vi "COMTRADE Read Data.vi"(0 "task in":T3={"file refnums"=[], "Data Object"=refnum, "config info"={"station_name"="", "rec_dev_id"="", "rev_year"=1999.0, "TT"=0, "##A"=0, "##D"=0, "analog channel info"=[], "status channel info"=[], "lf"=50.0, "nrates"=0, "samp info"=[], "initial timestamp"=timestamp(0 s since 1904-01-01), "trigger timestamp"=timestamp(0 s since 1904-01-01), "ft"=enum."Binary", "timemult"=1.0}, "public inf content"={"Source"="", "Record Type"=enum."Unknown", "Phase ID"="", "Event Description"="", "Device ID"="", "Distance of Fault"=-1.0, "Distance Unit"=enum."Miles", "Max_Current"=inf, "Min_Current"=-inf, "Max_Voltage"=inf, "Min_Voltage"=-inf, "EventNoteCount"=0, "Event Information"=[]}, "private inf content"=[], "internal buffers"={"start index"=1, "config to public inf"=enum."disabled", "static config info"="", "static file_des record inf"="", "static file_des channel inf"="", "public inf"="", "private inf"=""}} {"public inf content"."Event Information"."min sample number" max=9999999999; "public inf content"."Event Information"."max sample number" max=9999999999; "config info"."nrates" max=999; "config info"."status channel info"."Dn" min=1 max=999999; "config info"."analog channel info"."An" min=1 max=999999; "config info"."trigger timestamp" format="%<%H:%M:%S%6u\n%d/%m/%Y>T"; "config info"."initial timestamp" format="%<%H:%M:%S%6u\n%d/%m/%Y>T"; "config info"."##D" max=999999; "config info"."##A" max=999999; "config info"."TT" min=1 max=999999; "config info"."rev_year" min=1999.0 max=1999.0}, 11 "error in (no error)":errorcluster) -> (3 "number of sample rates":i32 min=0 max=999, 4 "task out":T3={"file refnums"=[], "Data Object"=refnum, "config info"={"station_name"="", "rec_dev_id"="", "rev_year"=1999.0, "TT"=0, "##A"=0, "##D"=0, "analog channel info"=[], "status channel info"=[], "lf"=50.0, "nrates"=0, "samp info"=[], "initial timestamp"=timestamp(0 s since 1904-01-01), "trigger timestamp"=timestamp(0 s since 1904-01-01), "ft"=enum."Binary", "timemult"=1.0}, "public inf content"={"Source"="", "Record Type"=enum."Unknown", "Phase ID"="", "Event Description"="", "Device ID"="", "Distance of Fault"=-1.0, "Distance Unit"=enum."Miles", "Max_Current"=inf, "Min_Current"=-inf, "Max_Voltage"=inf, "Min_Voltage"=-inf, "EventNoteCount"=0, "Event Information"=[]}, "private inf content"=[], "internal buffers"={"start index"=1, "config to public inf"=enum."disabled", "static config info"="", "static file_des record inf"="", "static file_des channel inf"="", "public inf"="", "private inf"=""}} {"public inf content"."Event Information"."min sample number" max=9999999999; "public inf content"."Event Information"."max sample number" max=9999999999; "config info"."nrates" max=999; "config info"."status channel info"."Dn" min=1 max=999999; "config info"."analog channel info"."An" min=1 max=999999; "config info"."trigger timestamp" format="%<%H:%M:%S%6u\n%d/%m/%Y>T"; "config info"."initial timestamp" format="%<%H:%M:%S%6u\n%d/%m/%Y>T"; "config info"."##D" max=999999; "config info"."##A" max=999999; "config info"."TT" min=1 max=999999; "config info"."rev_year" min=1999.0 max=1999.0}, 6 "sample rate information":T2(array[cluster]), 8 "analog data":T1(array[cluster]), 10 "digital data":digitaldata, 14 "timestamps":timestamp[](array[timestamp]), 15 "error out":errorcluster)   [LabVIEW 2014, in "NI_EP_COMTRADE.lvlib"]
doc: "Reads analog data and digital data from the specified .dat file. You must set <B>open mode</B> to Open (read only) in the COMTRADE Open VI to open the .inf file. Otherwise this VI returns an error."
uses:
  <vilib>/addons/Electrical Power/File IO/NI_EP_COMTRADE.lvlib
  <vilib>/addons/Electrical Power/File IO/COMTRADE/typedefs/ep_Task.ctl
  <vilib>/addons/Electrical Power/File IO/COMTRADE/typedefs/ep_Config Info.ctl
  <vilib>/addons/Electrical Power/File IO/COMTRADE/typedefs/ep_Analog Channel Info.ctl
  <vilib>/addons/Electrical Power/File IO/COMTRADE/typedefs/ep_Status Channel Info.ctl
  <vilib>/addons/Electrical Power/File IO/COMTRADE/typedefs/ep_File Format.ctl
  <vilib>/addons/Electrical Power/File IO/COMTRADE/typedefs/ep_Public Inf Content.ctl
  <vilib>/addons/Electrical Power/File IO/COMTRADE/typedefs/ep_Public Event Inf.ctl
  <vilib>/addons/Electrical Power/File IO/COMTRADE/typedefs/ep_Private Inf Content.ctl
  <vilib>/Analysis/1siggen.llb/Ramp Pattern by Samples.vi
  <vilib>/Platform/storage/Storage.llb/Get Property (Storage Refnums).vi
  <vilib>/Platform/storage/Storage.llb/Get Property (I32).vi
  <vilib>/Platform/storage/Storage.llb/Get Property (String).vi
  <vilib>/Platform/storage/Storage.llb/Get Property (SGL).vi
  <vilib>/Waveform/DTblOps.llb/DTbl Boolean Array to Digital.vi
  <vilib>/Analysis/NI_AALBase.lvlib
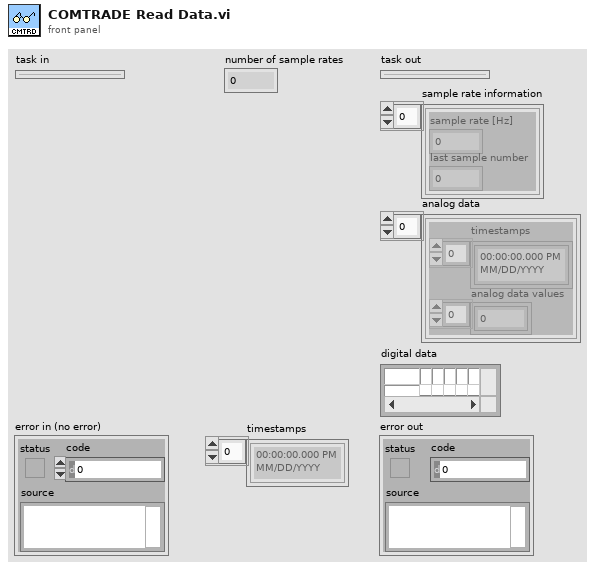
[diagram p1: front panel]
types:
  T1 = cluster{"timestamps":timestamp[], "analog data values":sgl[]}[]
  T2 = cluster{"sample rate [Hz]":sgl, "last sample number":u32}[]
  T3 = typedef "NI_EP_COMTRADE.lvlib/ep_Task.ctl" = cluster{"file refnums":refnum<file>[], "Data Object":refnum<k20>, "config info":T4, "public inf content":T8, "private inf content":T10, "internal buffers":cluster{"start index":u32, "config to public inf":enum16{"disabled", "enabled", "buffered"}, "static config info":string, "static file_des record inf":string, "static file_des channel inf":string, "public inf":string, "private inf":string}}
  T4 = typedef "NI_EP_COMTRADE.lvlib/ep_Config Info.ctl" = cluster{"station_name":string, "rec_dev_id":string, "rev_year":dbl, "TT":u32, "##A":u32, "##D":u32, "analog channel info":T5[], "status channel info":T6[], "lf":sgl, "nrates":u16, "samp info":cluster{"samp":sgl, "endsamp":u32}[], "initial timestamp":timestamp, "trigger timestamp":timestamp, "ft":T7, "timemult":sgl}
  T5 = typedef "NI_EP_COMTRADE.lvlib/ep_Analog Channel Info.ctl" = cluster{"An":u32, "ch_id":string, "ph":string, "ccbm":string, "uu":string, "a":sgl, "b":sgl, "skew":sgl, "min":i32, "max":i32, "primary":sgl, "secondary":sgl, "PS":enum16{"P", "S"}}
  T6 = typedef "NI_EP_COMTRADE.lvlib/ep_Status Channel Info.ctl" = cluster{"Dn":u32, "ch_id":string, "ph":string, "ccbm":string, "Y":bool}
  T7 = typedef "NI_EP_COMTRADE.lvlib/ep_File Format.ctl" = enum16{"ASCII", "Binary"}
  T8 = typedef "NI_EP_COMTRADE.lvlib/ep_Public Inf Content.ctl" = cluster{"Source":string, "Record Type":enum16{"Fault", "Unknown", "Misoperation", "Close", "Trip", "Reclose", "Power swing", "Simulation"}, "Phase ID":string, "Event Description":string, "Device ID":string, "Distance of Fault":dbl, "Distance Unit":enum16{"Miles", "Kilometers", "Percent of line", "Percent of setting", "Ohms"}, "Max_Current":dbl, "Min_Current":dbl, "Max_Voltage":dbl, "Min_Voltage":dbl, "EventNoteCount":u32, "Event Information":T9[]}
  T9 = typedef "NI_EP_COMTRADE.lvlib/ep_Public Event Inf.ctl" = cluster{"channel number":u32, "max value":dbl, "min value":dbl, "max sample number":u64, "min sample number":u64, "max sample text":string[], "min sample text":string[]}
  T10 = typedef "NI_EP_COMTRADE.lvlib/ep_Private Inf Content.ctl" = cluster{"Section Header":string, "Entry Names":string[], "Entry Values":string[]}[]
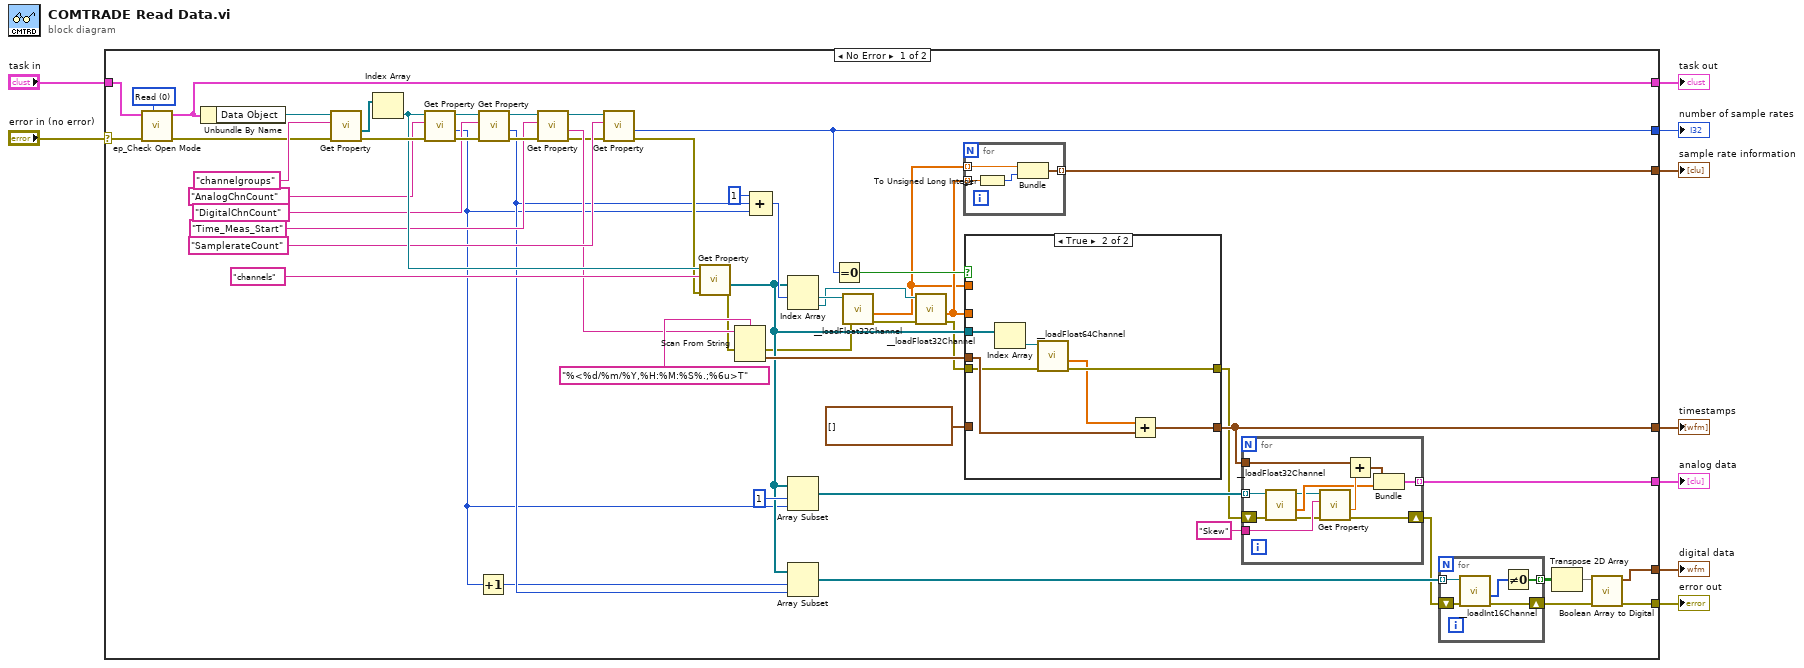
[diagram p0: block diagram]
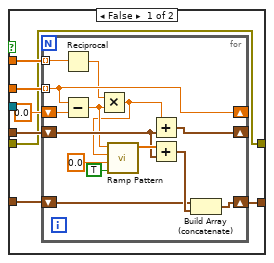
[diagram p2: hidden frame]
diagram:
  n1 = case shown="No Error" "error in (no error)" {
    selector: "error in (no error)" -> [w16 w114]
    tunnel: [w26 w114] -> w8
    tunnel: [w13 _] -> w7
    tunnel: "task in" -> [w14 _]
    tunnel: [w24 _] -> w5
    tunnel: [w56 _] -> w4
    tunnel: [w37 _] -> w3
    tunnel: [w36 _] -> w1
    tunnel: [w25 _] -> w2
    frame No Error {
      w17 = u16 0 items=["Read", "Write"] ("file type")
      n2 = call <vilib>:"ep_Check Open Mode.vi"("expected mode"=w17, "error in (no error)"=w16, "task in"=w14) -> ("error out"=w15:errorcluster, "task out"=w13:T3)  [unwired: 7 in]
      n3 = Unbundle By Name(w13) -> ("Data Object"=w64:refnum<k20>)
      n4 = call-poly <vilib>:"Get Property.vi"("error in (no error)"=w15, "Property name"="channelgroups", "storage refnum"=w64) -> ("error out"=w61:errorcluster, "Value"=w65:refnum<k20>[])  [unwired: 6 in, 1 out]
      n5 = Index Array(array=w65) -> (element=w52:refnum<k20>)  [unwired: 1 in]
      n6 = call-poly <vilib>:"Get Property.vi"("error in (no error)"=w61, "Property name"="AnalogChnCount", "storage refnum"=w52) -> ("error out"=w60:errorcluster, "Value"=w32:i32, "storage refnum out"=w59:refnum<k20>)  [unwired: 6 in]
      n7 = Increment(x=w32) -> (x+1=w33:i32)
      n8 = call-poly <vilib>:"Get Property.vi"("error in (no error)"=w60, "Property name"="DigitalChnCount", "storage refnum"=w59) -> ("error out"=w48:errorcluster, "Value"=w34:i32, "storage refnum out"=w49:refnum<k20>)  [unwired: 6 in]
      n9 = call-poly <vilib>:"Get Property.vi"("error in (no error)"=w48, "Property name"="Time_Meas_Start", "storage refnum"=w49) -> ("error out"=w11:errorcluster, "Value"=w44:string, "storage refnum out"=w10:refnum<k20>)  [unwired: 6 in]
      n10 = call-poly <vilib>:"Get Property.vi"("error in (no error)"=w11, "Property name"="SamplerateCount", "storage refnum"=w10) -> ("error out"=w42:errorcluster, "Value"=w24:i32)  [unwired: 6 in, 1 out]
      n11 = call-poly <vilib>:"Get Property.vi"("error in (no error)"=w42, "Property name"="channels", "storage refnum"=w52) -> ("error out"=w41:errorcluster, "Value"=w35:refnum<k20>[])  [unwired: 6 in, 1 out]
      n12 = Scan From String(format string="%<%d/%m/%Y,%H:%M:%S%.;%6u>T", input string=w44, error in=w41) -> (error out=w12:errorcluster, output 1=w43:timestamp)  [unwired: 2 in, 2 out]
      n13 = Compound Arithmetic op=ADD(1 ("value"), w34, w32) -> (w57:i32)
      n14 = Index Array(array=w35, index #1=w57) -> (element #1=w55:refnum<k20>, element #2=w53:refnum<k20>)  [unwired: 1 in]
      n15 = Array Subset(array=w35, index=1, length=w32) -> (w39:refnum<k20>[])
      n16 = Array Subset(array=w35, index=w33, length=w34) -> (w31:refnum<k20>[])
      n17 = Equal To 0?(x=w24) -> (x = 0?=w23:bool)
      n18 = call <vilib>:"__loadFloat32Channel.vi"("error in (no error)"=w12, "Data object in"=w55) -> ("error out"=w54:errorcluster, "Values"=w20:sgl[])  [unwired: 3 in, 1 out]
      n19 = call <vilib>:"__loadFloat32Channel.vi"("error in (no error)"=w54, "Data object in"=w53) -> ("error out"=w22:errorcluster, "Values"=w21:sgl[])  [unwired: 3 in, 1 out]
      n20 = for {
        tunnel: [w112] -> w56 mode=indexing
        tunnel: w20 -> [w111] mode=indexing
        tunnel: w21 -> [w110] mode=indexing
        n21 = To Unsigned Long Integer(number=w110) -> (unsigned 32bit integer=w113:u32)
        n22 = Bundle(w111, w113) -> (w112:cluster{sgl, u32})  [unwired: 1 in]
      }
      n23 = case shown="True" w23 {
        tunnel: w43 -> [w72 w92]
        tunnel: [w67 w91] -> w37
        tunnel: w35 -> [_ w90]
        tunnel: w22 -> [w66 w89]
        tunnel: [w66 w88] -> w18
        tunnel: w21 -> [w71 _]
        tunnel: w20 -> [w70 _]
        tunnel: timestamp[] [] ("element") -> [w68 _]
        frame False {
          n24 = for {
            shift-right: [w82] -> _
            shift-left: w72 -> [w78]
            tunnel: w71 -> [w84] mode=indexing
            tunnel: w70 -> [w86] mode=indexing
            shift-right: [w84] -> _
            shift-left: sgl 0.0 -> [w85]
            shift-right: [w76] -> w67
            shift-left: w68 -> [w74]
            n25 = Reciprocal(x=w86) -> (1/x=w83:sgl)
            n26 = Subtract(x=w84, y=w85) -> (x-y=w77:sgl)
            n27 = Multiply(x=w83, y=w77) -> (x*y=w73:sgl)
            n28 = call-poly <vilib>:"Ramp Pattern.vi"("exclude end?"=TRUE, "start"=0.0, "end"=w73, "samples"=w77) -> ("Ramp Pattern"=w79:dbl[])  [unwired: 6 in, 1 out]
            n29 = Add(x=w73, y=w78) -> (x+y=w82:timestamp)
            n30 = Add(x=w79, y=w78) -> (x+y=w75:timestamp[])
            n31 = Build Array (concatenate)(w74, w75) -> (w76:timestamp[])
          }
        }
        frame True {
          n32 = Index Array(array=w90) -> (element=w93:refnum<k20>)  [unwired: 1 in]
          n33 = call <vilib>:"__loadFloat64Channel.vi"("error in (no error)"=w89, "Data object in"=w93) -> ("error out"=w88:errorcluster, "Values"=w87:dbl[])  [unwired: 2 in, 2 out]
          n34 = Add(x=w87, y=w92) -> (x+y=w91:timestamp[])
        }
      }
      n35 = for {
        tunnel: w39 -> [w107] mode=indexing
        shift-right: [w103] -> w30
        shift-left: w18 -> [w108]
        tunnel: "Skew" ("Property name") -> [w109]
        tunnel: w37 -> [w105]
        tunnel: [w102] -> w36 mode=indexing
        n36 = call <vilib>:"__loadFloat32Channel.vi"("error in (no error)"=w108, "Data object in"=w107) -> ("error out"=w99:errorcluster, "Values"=w101:sgl[], "Data object out"=w100:refnum<k20>)  [unwired: 3 in]
        n37 = call-poly <vilib>:"Get Property.vi"("error in (no error)"=w99, "Property name"=w109, "storage refnum"=w100) -> ("error out"=w103:errorcluster, "Value"=w106:sgl)  [unwired: 6 in, 1 out]
        n38 = Add(x=w105, y=w106) -> (x+y=w104:timestamp[])
        n39 = Bundle(w104, "Values"=w101) -> (w102:cluster{timestamp[], "Values":sgl[]})  [unwired: 1 in]
      }
      n40 = for {
        tunnel: w31 -> [w98] mode=indexing
        tunnel: [w95] -> w29 mode=indexing
        shift-right: [w96] -> w27
        shift-left: w30 -> [w97]
        n41 = call <vilib>:"__loadInt16Channel.vi"("error in (no error)"=w97, "Data object in"=w98) -> ("error out"=w96:errorcluster, "Values"=w94:i16[])  [unwired: 2 in, 2 out]
        n42 = Not Equal To 0?(x=w94) -> (x != 0?=w95:bool[])
      }
      n43 = Transpose 2D Array(2D array=w29) -> (transposed array=w28:bool[][])
      n44 = call-poly <vilib>:"Boolean Array to Digital.vi"("error in (no error)"=w27, "boolean array"=w28) -> ("error out"=w26:errorcluster, "digital data"=w25:digitaldata)  [unwired: 8 in]
    }
    frame Error {
    }
  }
  "error out" <- w8
  "task out" <- w7
  "sample rate information" <- w4
  "number of sample rates" <- w5
  "digital data" <- w2
  "timestamps" <- w3
  "analog data" <- w1
